vi "test.vi"() -> ()   [LabVIEW 2023]
uses:
  Camera Imaqdx/Configuration/Camera Config Imaqdx/Camera Config Imaqdx.lvclass
  Camera Imaqdx/Camera Imaqdx.lvclass
  Camera Base.lvclass
  Camera Imaqdx/Stats.ctl
  Interfaces/IConfigure/IConfigure.lvclass
  D:/git/HAL/Camera Base/Camera Base.lvclass
  D:/git/HAL/Instrument/Instrument.lvclass
  D:/git/HAL/Interfaces/ICamera/ICamera.lvclass
  D:/git/HAL/Camera Imaqdx/Camera Imaqdx.lvclass
panel:
  out "Stats":T1
  out "Image":T2(plugin-control)
  out "error out":errorcluster
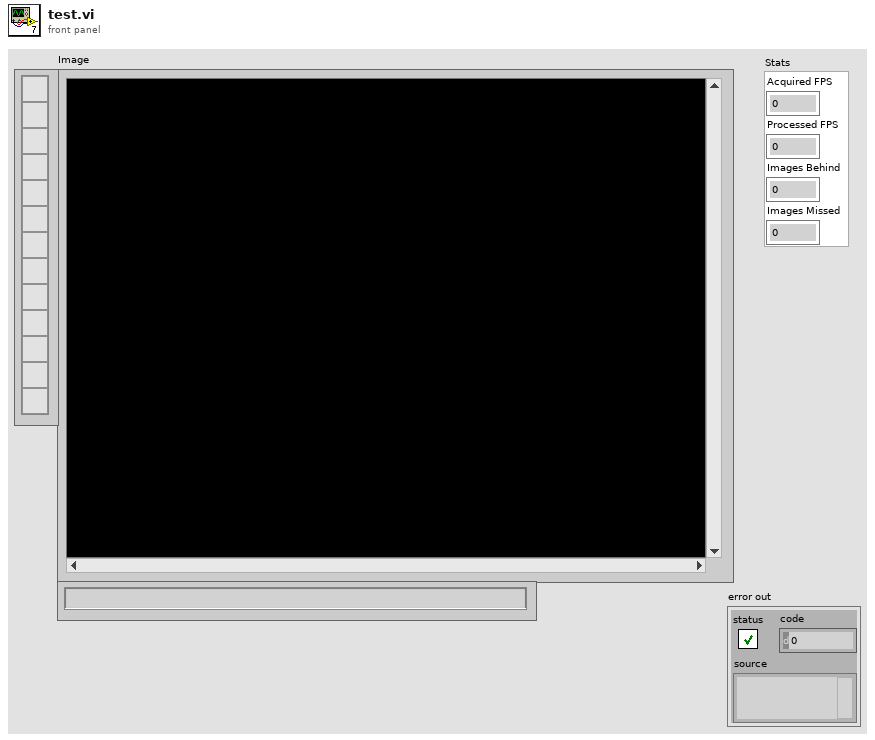
[diagram p1: front panel]
types:
  T1 = typedef "Camera Imaqdx.lvclass/Stats.ctl" = cluster{"Acquired FPS":dbl, "Processed FPS":dbl, "Images Behind":i32, "Images Missed":u32}
  T2 = typedef "IMAQ Image.ctl" = refnum<image>
  T3 = typedef "Camera Base.lvclass/Acquisition Stats.ctl" = cluster{"Acquired FPS":dbl, "Processed FPS":dbl, "Images Behind":u32, "Images Missed":u32}
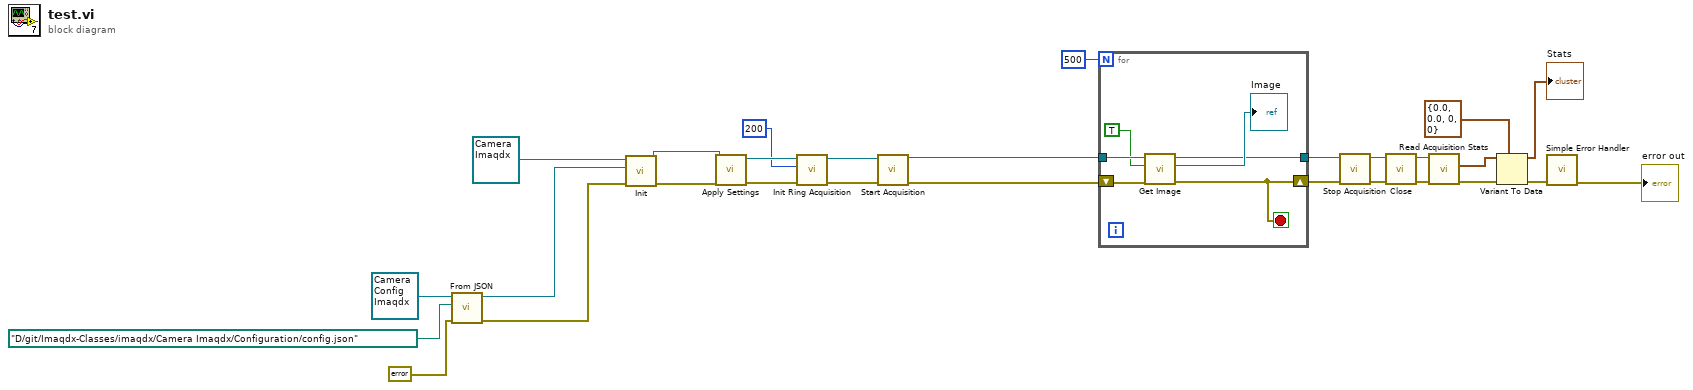
[diagram p0: block diagram]
diagram:
  n1 = call-dynamic "From JSON.vi"("error in"=errorcluster {"status"=FALSE, "code"=0, "source"=""} ("error in (no error)"), "JSON Config"=path "D:/git/Imaqdx-Classes/imaqdx/Camera Imaqdx/Configuration/config.json", "Camera Config Imaqdx in"=refnum<class "Camera Config Imaqdx.lvclass"> refnum ("Cameras.lvlib:Camera Config Imaqdx.lvclass")) -> ("error out"=w25:errorcluster, "Camera Config Imaqdx out"=w28:refnum<class "Camera Config Imaqdx.lvclass">)  [unwired: 7 in]
  n2 = call-dynamic "Init.vi"("error in (no error)"=w25, "IConfigure"=w28, "Camera Base in"=refnum<class "Camera Imaqdx.lvclass"> refnum ("Cameras.lvlib:Camera Imaqdx.lvclass")) -> ("error out"=w24:errorcluster, "Camera Base out"=w23:refnum<class "Camera Imaqdx.lvclass">)  [unwired: 7 in]
  n3 = call-dynamic "Apply Settings.vi"("error in (no error)"=w24, "Camera Base in"=w23) -> ("error out"=w21:errorcluster, "Camera Base out"=w18:refnum<class "Camera Imaqdx.lvclass">)  [unwired: 8 in]
  n4 = call-dynamic "Init Ring Acquisition.vi"("error in (no error)"=w21, "Ring Buffer Size"=u32 200, "Camera Imaqdx in"=w18) -> ("error out"=w19:errorcluster, "Camera Imaqdx out"=w17:refnum<class "Camera Imaqdx.lvclass">)  [unwired: 7 in]
  n5 = call-dynamic "Start Acquisition.vi"("error in"=w19, "Camera Imaqdx in"=w17) -> ("error out"=w15:errorcluster, "Camera Imaqdx out"=w13:refnum<class "Camera Imaqdx.lvclass">)  [unwired: 8 in]
  n6 = for {
    N: 500 -> [_]
    tunnel: w13 -> [w34]
    shift-right: [w29] -> w11
    shift-left: w15 -> [w33]
    tunnel: [w31] -> w7
    stop <- w29 stop-if-true
    n7 = call-dynamic "Get Image.vi"("error in"=w33, "Calc Stats?"=TRUE, "Camera Imaqdx in"=w34) -> ("error out"=w29:errorcluster, "Image out"=→"Image":T2, "Camera Imaqdx out"=w31:refnum<class "Camera Imaqdx.lvclass">)  [unwired: 6 in]
  }
  n8 = call-dynamic "Stop Acquisition.vi"("error in"=w11, "Camera Imaqdx in"=w7) -> ("error out"=w8:errorcluster, "Camera Imaqdx out"=w5:refnum<class "Camera Imaqdx.lvclass">)  [unwired: 8 in]
  n9 = call-dynamic "Close.vi"("error in (no error)"=w8, "Camera Base in"=w5) -> ("error out"=w6:errorcluster, "Camera Base out"=w4:refnum<class "Camera Imaqdx.lvclass">)  [unwired: 8 in]
  n10 = call "Read Acquisition Stats.vi"("error in (no error)"=w6, "Camera Base in"=w4) -> ("error out"=w10:errorcluster, "Acquisition Stats"=w9:T3)  [unwired: 7 in, 1 out]
  n11 = Variant To Data(error in=w10, type=T1 {"Acquired FPS"=0.0, "Processed FPS"=0.0, "Images Behind"=0, "Images Missed"=0} ("Stats"), Variant=w9) -> (data=→"Stats":T1, error out=w1:errorcluster)
  n12 = call <vilib>:"Simple Error Handler.vi"("error in (no error)"=w1) -> ("error out"=→"error out":errorcluster)  [unwired: 4 in, 4 out]
